vi "Get SubNumber+.vi"(8 "Error In":errorcluster, 11 "reference in":refnum<class "OD Entry.lvclass">) -> (0 "Error Out":errorcluster, 1 "Defined?":bool, 2 "SubNumber":u8 format="%.0x", 3 "reference out":refnum<class "OD Entry.lvclass">)   [LabVIEW 2019, in "Electronic Datasheet.lvlib" / "OD Entry.lvclass"]
uses:
  OD Entry.lvclass
  Object Type/Object Type Base.lvclass
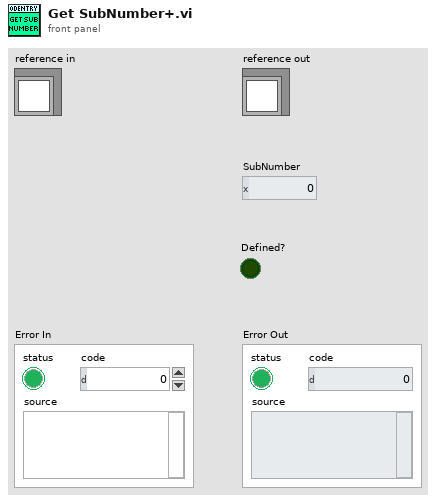
[diagram p1: front panel]
types:
  T1 = typedef "Electronic Datasheet.lvlib/OD Entry.lvclass/ObjectAttributes.ctl" = cluster{"Index":u16, "ObjectType":refnum<class "Object Type Base.lvclass">, "Denotation":string, "Count":u8, "ObjExtend":u8, "Label":string, "Description":string, "PDO Mapping Type":T2, "Sub-Entries":map{u8, refnum<class "OD Sub-Entry.lvclass">}}
  T2 = typedef "Electronic Datasheet.lvlib/PDO Mapping Type.ctl" = enum16{"no", "optional", "RPDO", "TPDO", "UNKNOWN"}
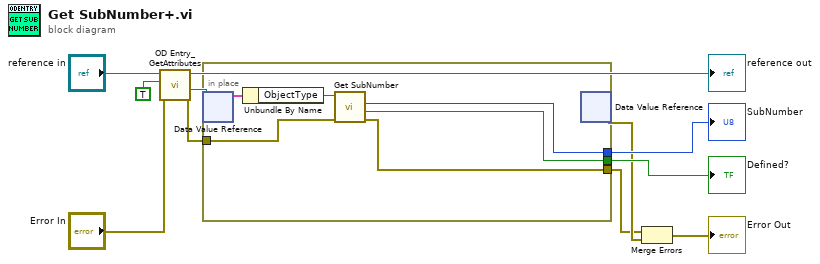
[diagram p0: block diagram]
diagram:
  n1 = call "OD Entry_GetAttributes.vi"("Error In"="Error In", "OnlyGetDvrReference(False)"=TRUE, "reference in"="reference in") -> ("Error Out"=w2:errorcluster, "DataRef"=w3:refnum<data-value>, "reference out"=→"reference out":refnum<class "OD Entry.lvclass">)  [unwired: 5 in, 1 out]
  n2 = in-place {
    in-place-border: w2 -> [w15]
    in-place-border: [w12] -> w1
    in-place-border: [w14] -> w7
    in-place-border: [w13] -> w6
    n3 = in-place-dvr #1(w3) -> (w16:T1)  [unwired: 1 out]
    n4 = Unbundle By Name(w16) -> ("ObjectType"=w17:refnum<class "Object Type Base.lvclass">)
    n5 = call-dynamic "Get SubNumber.vi"("error in"=w15, "Object Type in"=w17) -> ("error out"=w12:errorcluster, "Set?"=w13:bool, "SubNumber"=w14:u8)  [unwired: 6 in, 1 out]
    n6 = in-place-dvr #1() -> (w5:errorcluster)  [unwired: 1 in, 1 out]
  }
  "Defined?" <- w6
  "SubNumber" <- w7
  n7 = Merge Errors(w1, w5) -> (→"Error Out":errorcluster)
